vi "Configure Trigger (Glitch).vi"(4 "Trigger Level (0.0 V)":dbl, 5 "Polarity (0: Positive)":i32(ring) items=["Positive", "Negative"], 6 "Pulse Width High Threshold (1.0 S)":dbl=1.0, 7 "Pulse Width Low Threshold (1.0 S)":dbl=1.0, 8 "error in (no error)":errorcluster, 9 "Qualifier (0: Maximum Limit)":i32(ring) items=["Maximum Limit", "Minimum Limit", "Range"], 10 "Trigger Source (0: Channel 1)":i32(ring) items=["Channel 1"=0, "Channel 2"=1, "Channel 3"=2, "Channel 4"=3, "D0"=13, "D1"=14, "D2"=15, "D3"=16, "D4"=17, "D5"=18, "D6"=19, "D7"=20, "D8"=21, "D9"=22, "D10"=23, "D11"=24, "D12"=25, "D13"=26, "D14"=27, "D15"=28], 11 "VISA resource name":refnum<visa-resource-name>) -> (0 "error out":errorcluster, 3 "VISA resource name out":refnum<visa-resource-name>)   [LabVIEW 2015, in "Agilent 2000 3000 X-Series.lvlib"]
doc: "Configures the glitch trigger mode."
uses:
  <instrlib>/Agilent 2000 3000 X-Series/Agilent 2000 3000 X-Series.lvlib
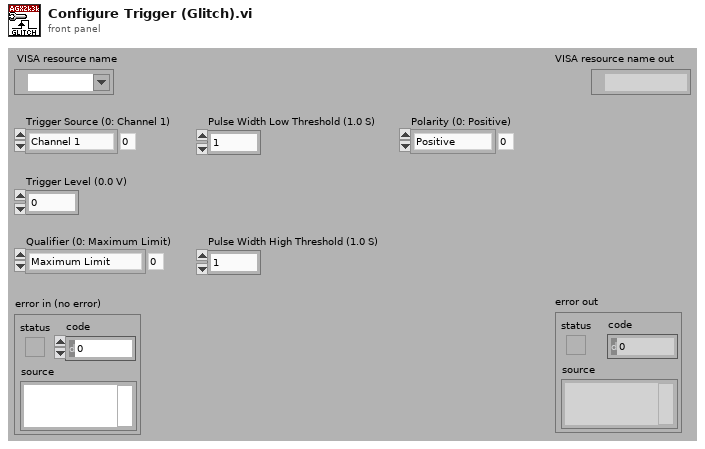
[diagram p1: front panel]
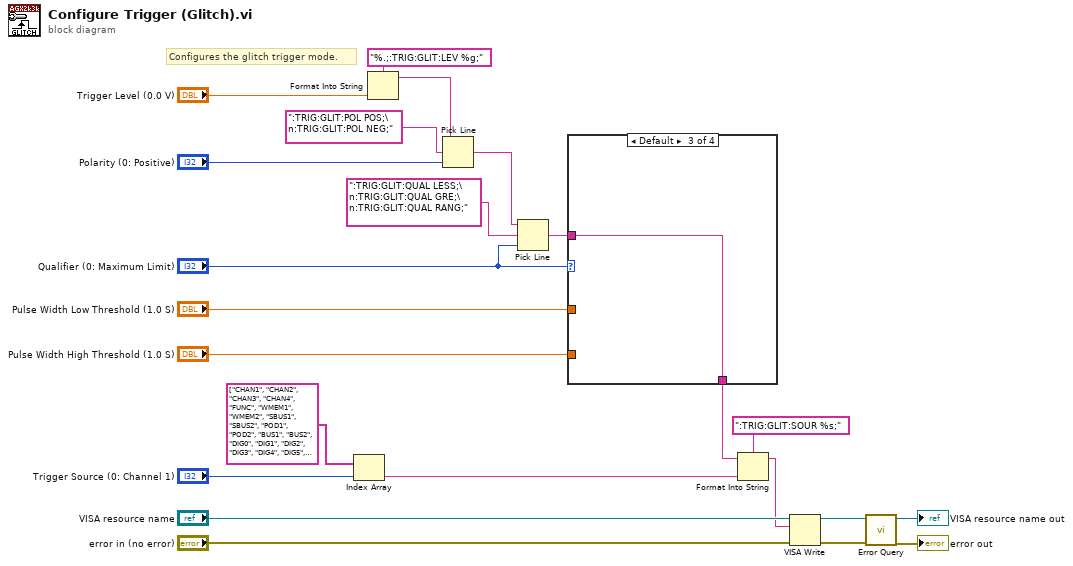
[diagram p0: block diagram]
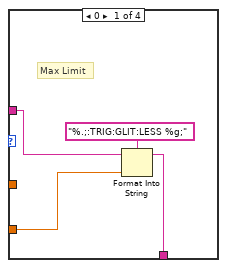
[diagram p2: hidden frame]
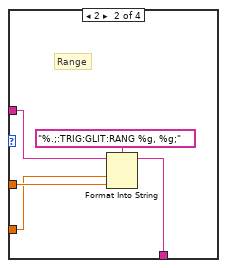
[diagram p3: hidden frame]
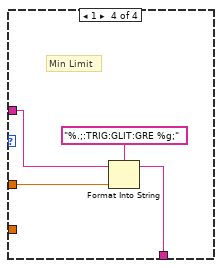
[diagram p4: hidden frame]
diagram:
  # "Configures the glitch trigger mode."
  n1 = Index Array(array=string[] ["CHAN1", "CHAN2", "CHAN3", "CHAN4", "FUNC", "WMEM1", "WMEM2", "SBUS1", "SBUS2", "POD1", "POD2", "BUS1", "BUS2", "DIG0", "DIG1", "DIG2", "DIG3", "DIG4", "DIG5", "DIG6", "DIG7", "DIG8", "DIG9", "DIG10", "DIG11", "DIG12", "DIG13", "DIG14", "DIG15", "EXT", "LINE", "WGEN"], index="Trigger Source (0: Channel 1)") -> (element=w1:string)
  n2 = Format Into String(format string="%.;:TRIG:GLIT:LEV %g;", "Trigger Level (0.0 V)") -> (resulting string=w19:string)  [unwired: 2 in, 1 out]
  n3 = Pick Line(string ("")=w19, multi-line string=":TRIG:GLIT:POL POS;\n:TRIG:GLIT:POL NEG;", line index="Polarity (0: Positive)") -> (output string=w17:string)
  n4 = Pick Line(string ("")=w17, multi-line string=":TRIG:GLIT:QUAL LESS;\n:TRIG:GLIT:QUAL GRE;\n:TRIG:GLIT:QUAL RANG;", line index="Qualifier (0: Maximum Limit)") -> (output string=w7:string)
  n5 = case shown="Default" "Qualifier (0: Maximum Limit)" {
    tunnel: "Pulse Width Low Threshold (1.0 S)" -> [_ w31 _ w37]
    tunnel: "Pulse Width High Threshold (1.0 S)" -> [w26 w30 _ _]
    tunnel: w7 -> [w25 w29 w33 w35]
    tunnel: [w24 w28 w33 w34] -> w6
    frame 0 {
      # "Max Limit"
      n6 = Format Into String(format string="%.;:TRIG:GLIT:LESS %g;", initial string=w25, w26) -> (resulting string=w24:string)  [unwired: 1 in, 1 out]
    }
    frame 2 {
      # "Range"
      n7 = Format Into String(format string="%.;:TRIG:GLIT:RANG %g, %g;", initial string=w29, w30, w31) -> (resulting string=w28:string)  [unwired: 1 in, 1 out]
    }
    frame Default {
    }
    frame 1 {
      # "Min Limit"
      n8 = Format Into String(format string="%.;:TRIG:GLIT:GRE %g;", initial string=w35, w37) -> (resulting string=w34:string)  [unwired: 1 in, 1 out]
    }
  }
  n9 = Format Into String(format string=":TRIG:GLIT:SOUR %s;", initial string=w6, w1) -> (resulting string=w4:string)  [unwired: 1 in, 1 out]
  n10 = VISA Write(VISA resource name="VISA resource name", write buffer=w4, error in (no error)="error in (no error)") -> (VISA resource name out=w14:refnum<visa-resource-name>, error out=w13:errorcluster)  [unwired: 1 out]
  n11 = call <instrlib>:"Error Query.vi"("error in (no error)"=w13, "VISA resource name"=w14) -> ("error out"=→"error out":errorcluster, "VISA resource name out"=→"VISA resource name out":refnum<visa-resource-name>)  [unwired: 8 out]
